vi "transmisor PSK.vi"() -> ()   [LabVIEW 2016]
uses:
  <vilib>/addons/Modulation/Digital/Support/Controls/Pack Bits Parameters.ctl
  <vilib>/addons/Modulation/Analog/support/mod_Set Error Source.vi
  <vilib>/addons/Modulation/Digital/Support/Common/Validators/mod_Generate Filter Coefficients Validate.vi
  <vilib>/addons/Modulation/Digital/General/subVIs/mod_Generate Filter Coefficients.vi
  <vilib>/addons/Modulation/Digital/General/MT Generate PSK System Parameters(M).vi
  <instrlib>/niUSRP/niUSRP Write Tx Data (CDB Cluster).vi
  <vilib>/addons/Modulation/niDMT.lvlib
panel:
  out "Cola":i8[](array[numeric])
  in  "Cola":u32=10 format="%b"
  out "Header+Bit+Cola":i16[](array[numeric])
  out "Header":i8[](array[numeric])
  in  "Header":u32=10 format="%b"
  out "session handle out":refnum<k15>
  in  "device names":refnum<k15>
  out "input bit stream":i8[](array[numeric])
  out "Frame Size [samples]":i32=4092
  out "Constellation Graph":T1(graph) caption="Tx Signal Constellation"
  in  "filter parameters":T2={"Alpha"=0.5, "Filter Length"=6, "TX Filter"=enum."Root Raised Cos"} {"Alpha" format="%.2f"}
  out "symbols out":cdb[](array[numeric]) format="%.2f"
  out "Symbol Rate\n[symbols/sec]":dbl=500000.0 format="%#.6p"
  in  "Bit":u32=10 format="%b"
  in  "stop":bool
  in  "Tx Parameters":T3={"Tx IQ Sampling\nRate [s/sec]"=400000.0, "Tx Frequency [Hz]"=915000000.0, "Tx Gain [dB]"=0.0, "Tx Antenna"="TX1"} {"Tx Gain [dB]" format="%#.6p"; "Tx Frequency [Hz]" format="%#.6p"; "Tx IQ Sampling\nRate [s/sec]" format="%#.6p"}
  out "Actual Tx Parameters":T3={"Tx IQ Sampling\nRate [s/sec]"=400000.0, "Tx Frequency [Hz]"=915000000.0, "Tx Gain [dB]"=0.0, "Tx Antenna"="TX1"} {"Tx Gain [dB]" format="%#.6p"; "Tx Frequency [Hz]" format="%#.6p"; "Tx IQ Sampling\nRate [s/sec]" format="%#.6p"}
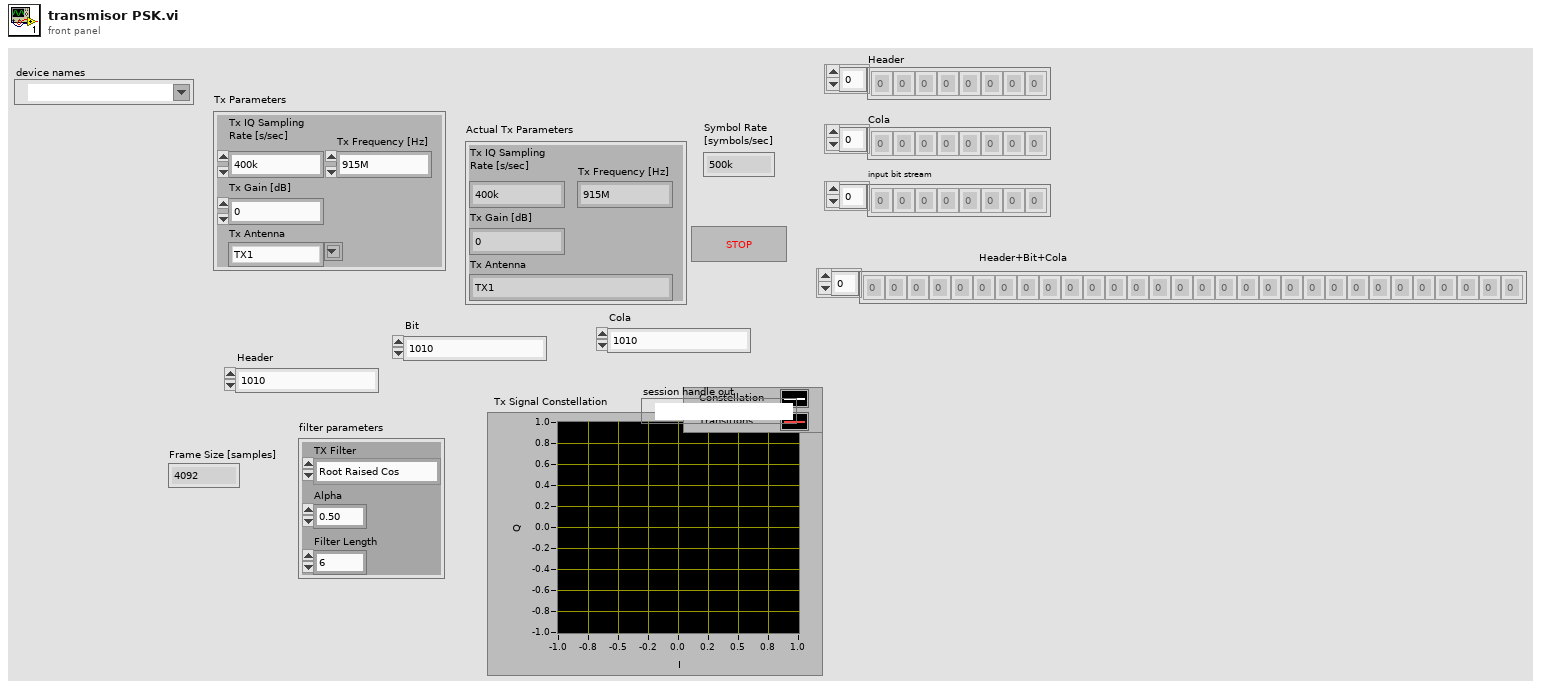
[diagram p1: front panel]
types:
  T1 = cluster{"constellation":dbl[], "oversampled data":dbl[]}[]
  T2 = cluster{"Alpha":dbl, "Filter Length":i32, "TX Filter":enum16{"none", "Raised Cosine", "Root Raised Cos", "Gaussian"}}
  T3 = cluster{"Tx IQ Sampling\nRate [s/sec]":dbl, "Tx Frequency [Hz]":dbl, "Tx Gain [dB]":dbl, "Tx Antenna":string}
  T4 = typedef "niDMT.lvlib/Pack Bits Parameters.ctl" = enum16{"Unsigned", "Signed"}
  T5 = enum16{"FSK", "PSK", "QAM", "MSK", "PAM", "ASK", "CPM"}
  T6 = enum16{"none", "Raised Cosine", "Root Raised Cos", "Gaussian"}
  T7 = cluster{"samples per symbol (16)":i32, "symbol map":cdb[], "differential PSK":enum16{"disable", "enable"}, "PSK type":u16}
  T8 = typedef "niAMT.lvlib/Complex Data Waveform.ctl" = cluster{"t0":dbl, "dt":dbl, "Y":cdb[]}
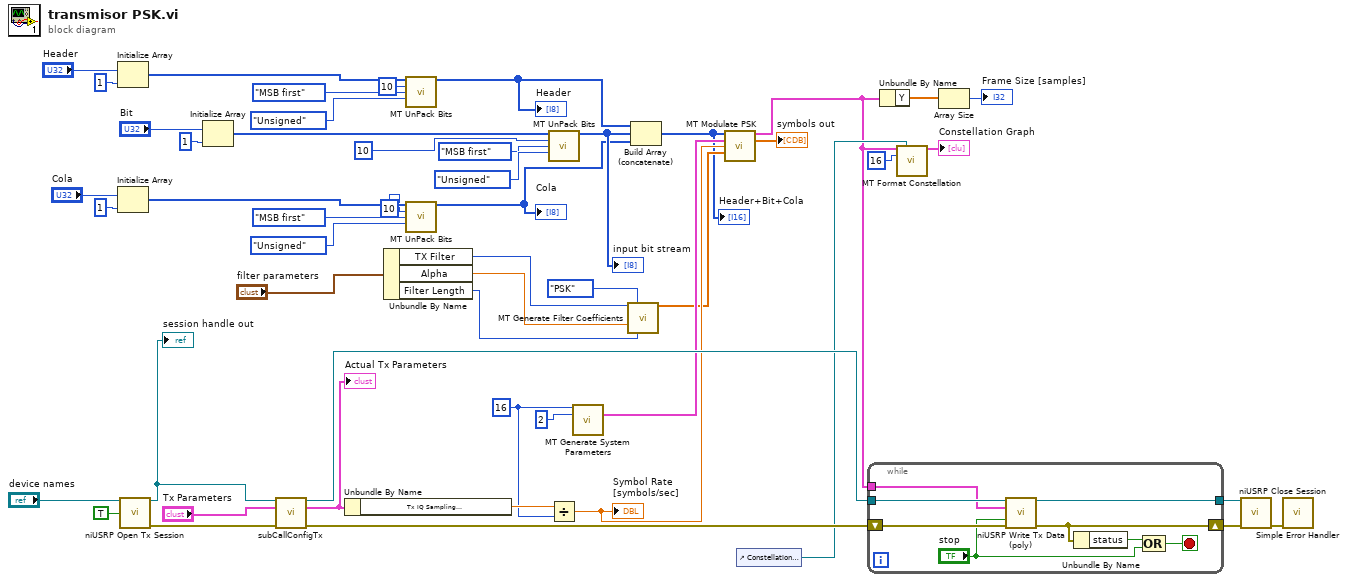
[diagram p0: block diagram]
diagram:
  w21 = 16 ("samples per symbol (16)")
  n1 = Initialize Array("Header", 1 ("dimension size")) -> (w6:u32[])
  n2 = Initialize Array("Cola", 1 ("dimension size")) -> (w4:u32[])
  n3 = call <instrlib>:"niUSRP Open Tx Session.vi"("device names"="device names", "reset"=TRUE) -> ("session handle out"=w19:refnum<k15>, "error out"=w49:errorcluster)  [unwired: 12 in]
  "session handle out" <- w19
  n4 = Initialize Array("Bit", 1 ("dimension size")) -> (w3:u32[])
  n5 = call "subCallConfigTx.vi"("session handle"=w19, "Tx Parameters"="Tx Parameters", "error in"=w49) -> ("session handle out"=w44:refnum<k15>, "Actual Tx Parameters"=w50:T3, "error out"=w43:errorcluster)  [unwired: 10 in]
  "Actual Tx Parameters" <- w50
  n6 = Unbundle By Name(w50) -> ("Tx IQ Sampling\nRate [s/sec]"=w39:dbl)
  n7 = Unbundle By Name("filter parameters") -> ("TX Filter"=w33:T6, "Alpha"=w32:dbl, "Filter Length"=w31:i32)
  n8 = call <vilib>:"MT UnPack Bits.vi"("input integers"=w6, "bits per integer"=10, "packed bit order"=enum16{"MSB first", "LSB first"}."MSB first", "integer format"=Pack_Bits_Parameters."Unsigned") -> ("output bit stream"=w14:i8[])  [unwired: 10 in, 1 out]
  "Header" <- w14
  n9 = call <vilib>:"MT UnPack Bits.vi"("input integers"=w4, "bits per integer"=10, "packed bit order"=enum16{"MSB first", "LSB first"}."MSB first", "integer format"=Pack_Bits_Parameters."Unsigned") -> ("output bit stream"=w7:i8[])  [unwired: 10 in, 1 out]
  "Cola" <- w7
  n10 = call <vilib>:"MT UnPack Bits.vi"("input integers"=w3, "bits per integer"=10, "packed bit order"=enum16{"MSB first", "LSB first"}."MSB first", "integer format"=Pack_Bits_Parameters."Unsigned") -> ("output bit stream"=w13:i8[])  [unwired: 10 in, 1 out]
  "input bit stream" <- w13
  n11 = Divide(x=w39, y=w21) -> (x/y=w38:dbl)
  "Symbol Rate\n[symbols/sec]" <- w38
  n12 = call-poly <vilib>:"MT Generate System Parameters.vi"("samples per symbol (16)"=w21, "M-PSK (4)"=2) -> ("PSK system parameters"=w41:T7)  [unwired: 11 in, 2 out]
  n13 = call <vilib>:"MT Generate Filter Coefficients.vi"("pulse shaping filter (none)"=w33, "modulation type"=T5."PSK", "filter parameter"=w32, "filter length (symbols)"=w31) -> ("pulse shaping filter coefficients"=w36:dbl[])  [unwired: 9 in, 2 out]
  n14 = Build Array (concatenate)(w14, w13, w7) -> (w12:i8[])
  "Header+Bit+Cola" <- w12
  n15 = call <vilib>:"MT Modulate PSK.vi"("input bit stream"=w12, "PSK system parameters"=w41, "symbol rate (Hz)"=w38, "pulse shaping filter coefficients"=w36) -> ("output complex waveform"=w26:T8, "symbols out"=→"symbols out":cdb[])  [unwired: 9 in, 1 out]
  n16 = control-ref of="Constellation Graph"() -> (w30:refnum<vi>)
  n17 = while {
    tunnel: [w57] -> w46
    tunnel: w44 -> [w59]
    shift-right: [w53] -> w47
    shift-left: w43 -> [w58]
    tunnel: w26 -> [w52]
    stop <- w56 stop-if-true
    n18 = call-poly <instrlib>:"niUSRP Write Tx Data (poly).vi"("session handle"=w59, "data"=w52, "end of data?"="stop", "error in (no error)"=w58) -> ("session handle out"=w57:refnum<k15>, "error out"=w53:errorcluster)  [unwired: 10 in]
    n19 = Unbundle By Name(w53) -> ("status"=w55:bool)
    n20 = Compound Arithmetic op=OR(w55, "stop") -> (w56:bool)
  }
  n21 = Unbundle By Name(w26) -> ("Y"=w25:cdb[])
  n22 = call <vilib>:"MT Format Constellation.vi"("waveform"=w26, "constellation reference"=w30, "samples per symbol"=16) -> ("constellation graph"=→"Constellation Graph":T1)  [unwired: 11 in, 1 out]
  n23 = Array Size(array=w25) -> (size(s)=→"Frame Size [samples]":i32)
  n24 = call <instrlib>:"niUSRP Close Session.vi"("session handle"=w46, "error in (no error)"=w47) -> ("error out"=w45:errorcluster)  [unwired: 13 in]
  n25 = call <vilib>:"Simple Error Handler.vi"("error in (no error)"=w45) -> ()  [unwired: 4 in, 5 out]
